vi "16转10.vi"(1 "字符串":string) -> (0 "字符串 2":string)   [LabVIEW 2015]
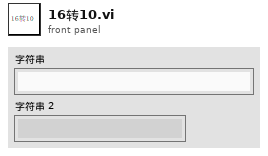
[diagram p1: front panel]
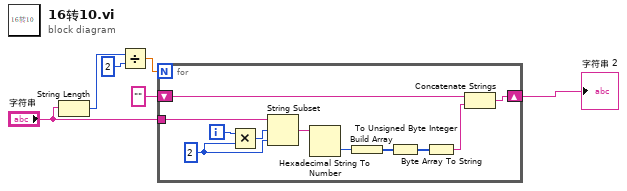
[diagram p0: block diagram]
diagram:
  n1 = String Length(string="字符串") -> (length=w6:i32)
  n2 = Divide(x=w6, y=2) -> (x/y=w4:dbl)
  n3 = for {
    N: w4 -> [_]
    tunnel: "字符串" -> [w15]
    shift-right: [w16] -> w1
    shift-left: "" ("字符串") -> [w17]
    i -> [w14]
    w13 = 2 ("y")
    n4 = Multiply(x=w14, y=w13) -> (x*y=w12:i32)
    n5 = String Subset(string=w15, offset (0)=w12, length (rest)=w13) -> (substring=w11:string)
    n6 = Hexadecimal String To Number(string=w11) -> (number=w10:u32)  [unwired: 2 in, 1 out]
    n7 = Build Array(w10) -> (w9:u32[])
    n8 = To Unsigned Byte Integer(number=w9) -> (unsigned 8bit integer=w8:u8[])
    n9 = Byte Array To String(unsigned byte array=w8) -> (string=w7:string)
    n10 = Concatenate Strings(w17, w7) -> (w16:string)
  }
  "字符串 2" <- w1
